vi "Get Selection from TreeBrowserWF.vi"(8 "error in (no error)":errorcluster, 10 "Input Channels":variant, 11 ".NET Refnum in":refnum<k24>) -> (0 "error out":errorcluster, 3 "Input Channel Selections":T1[](array[typedef]) {"Data Type" items=["Signed", "Unsigned", "IEEE Float"]})   [LabVIEW 2016, in "LIN Frame Protection Addon System Explorer.lvlib"]
uses:
  LIN Frame Protection Addon System Explorer.lvlib
  Shared/Types/InputChannelConfiguration.ctl
  NationalInstruments.VeriStand.SystemStorageUI
  NationalInstruments.VeriStand.SystemStorage
  Shared/LIN Frame Protection Addon Shared.lvlib
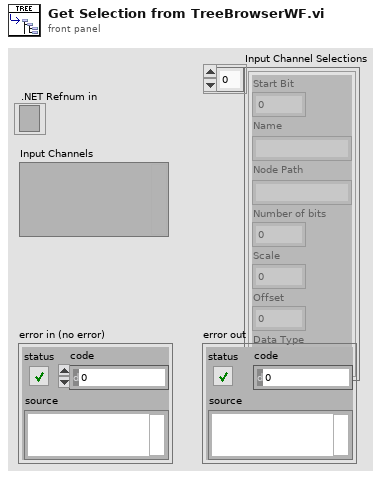
[diagram p1: front panel]
types:
  T1 = typedef "LIN Frame Protection Addon Shared.lvlib/InputChannelConfiguration.ctl" = cluster{"Start Bit":i32, "Name":string, "Node Path":string, "Number of bits":i32, "Scale":dbl, "Offset":dbl, "Data Type":u32}
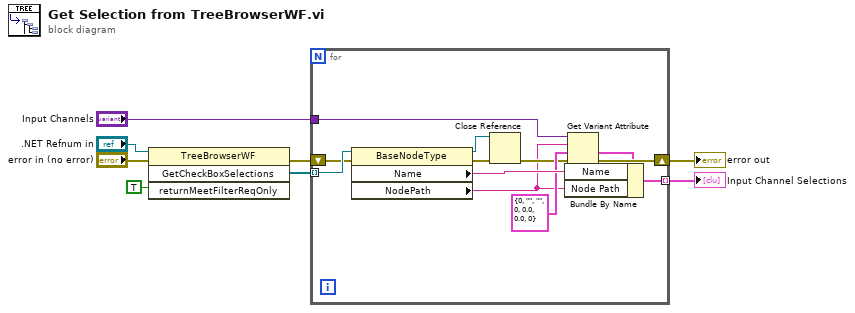
[diagram p0: block diagram]
diagram:
  n1 = invoke class="TreeBrowserWF" method="GetCheckBoxSelections"(reference=".NET Refnum in", error in="error in (no error)", "returnMeetFilterReqOnly"=TRUE) -> (error out=w5:errorcluster, "GetCheckBoxSelections"=w4:refnum<k24>[])  [unwired: 1 in, 2 out]
  n2 = for {
    tunnel: w4 -> [w20] mode=indexing
    shift-right: [w16] -> w6
    shift-left: w5 -> [w19]
    tunnel: [w17] -> w7 mode=indexing
    tunnel: "Input Channels" -> [w15]
    n3 = property class="BaseNodeType"(reference=w20, error in=w19) -> (reference out=w10:refnum<k24>, error out=w12:errorcluster, "Name"=w18:string, "NodePath"=w9:string)
    n4 = Close Reference(reference=w10, error in (no error)=w12) -> (error out=w11:errorcluster)
    n5 = Get Variant Attribute(Variant=w15, name=w9, default value (empty Variant)=T1 {"Start Bit"=0, "Name"="", "Node Path"="", "Number of bits"=0, "Scale"=0.0, "Offset"=0.0, "Data Type"=0} ("MonitoredChannelSettings"), error in=w11) -> (value=w14:T1, error out=w16:errorcluster)  [unwired: 2 out]
    n6 = Bundle By Name(cluster=w14, "Name"=w18, "Node Path"=w9) -> (w17:T1)
  }
  "Input Channel Selections" <- w7
  "error out" <- w6
